vi "configureHWError.vi"(8 "error in (no error)":errorcluster, 11 "AtomChipHWC in":refnum<class "AtomChipHWC.lvclass">) -> (0 "error out":errorcluster, 2 "error":bool, 3 "AtomChipHWC out":refnum<class "AtomChipHWC.lvclass">)   [LabVIEW 2009, in "Hardware.lvlib" / "HWControllers.lvlib" / "AtomChipHWC.lvclass"]
uses:
  AtomChipHWC.lvclass
  AtomChipHWC.lvclass/AtomChipHWC.ctl
  Channels/Digital/DigitalOutput.lvclass
  Channels/VoltOutput/AnalogOutput.lvclass
  Channels/DDSOutput/Generic/DDSOutput.lvclass
  Network Controllers/CameraNetworkController/CameraNetworkController.lvclass
  HWController.lvclass
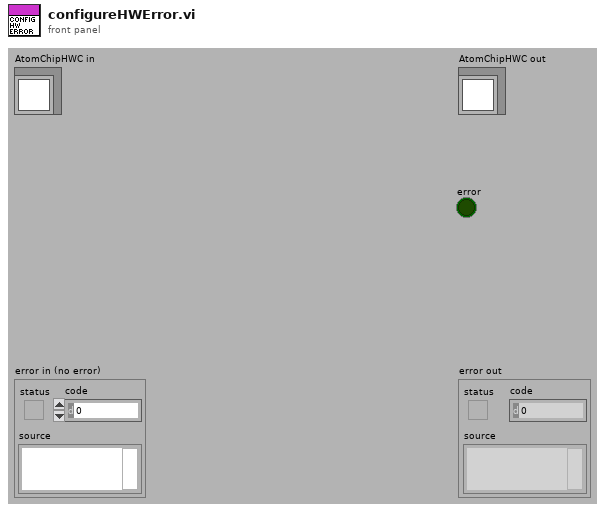
[diagram p1: front panel]
types:
  T1 = enum16{"Ready", "Compiling", "Configured", "Running", "Stopping", "Unresolved Error"}
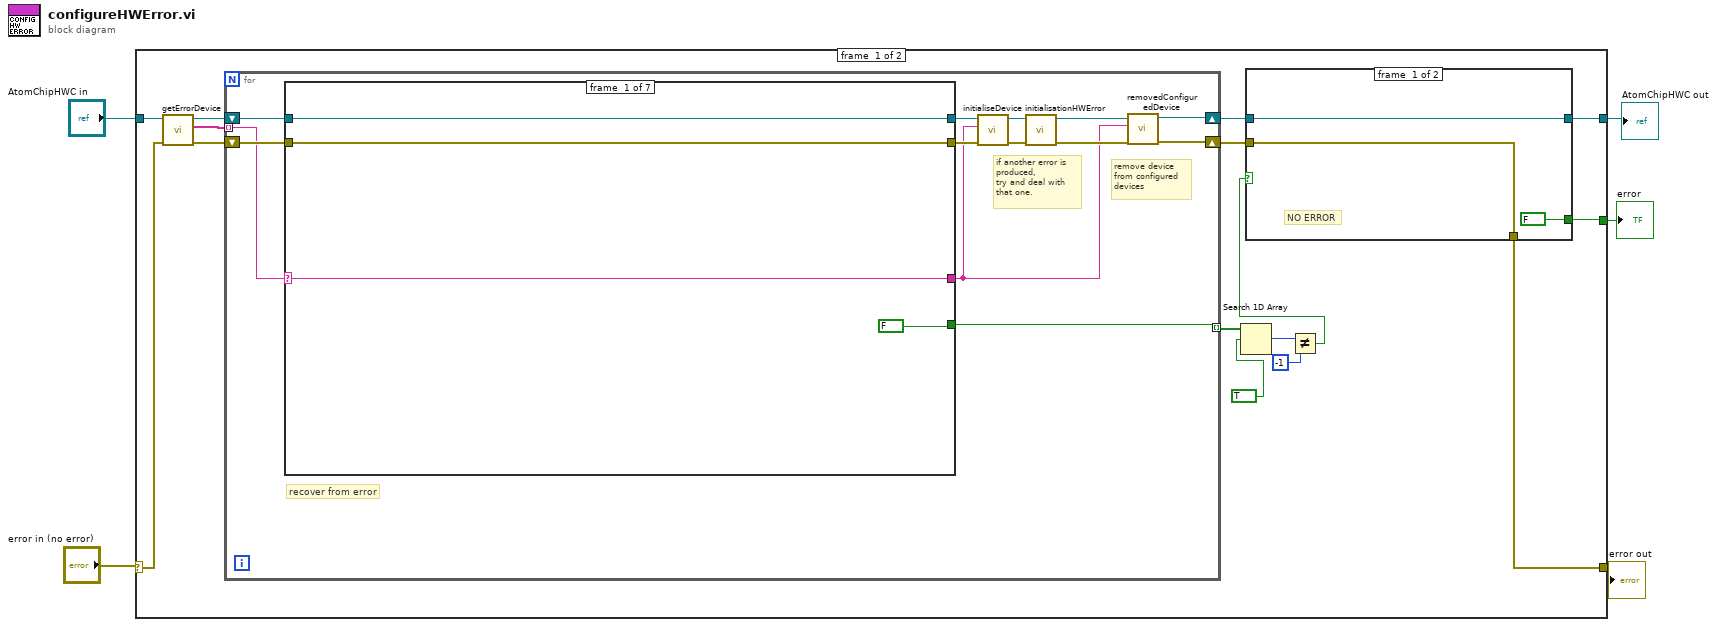
[diagram p0: block diagram]
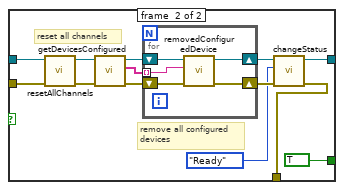
[diagram p2: hidden frame]
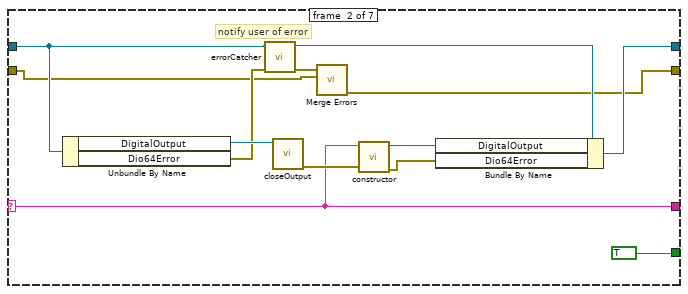
[diagram p3: hidden frame]
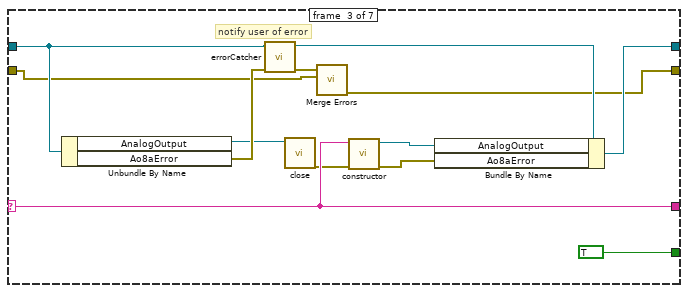
[diagram p4: hidden frame]
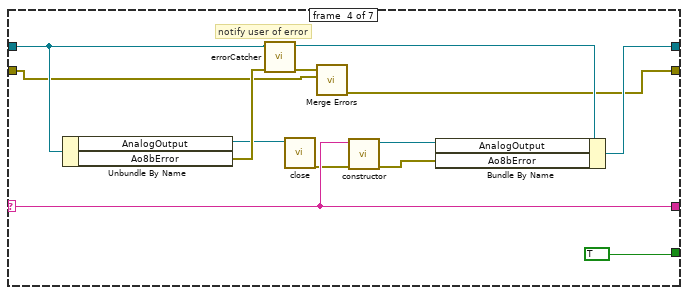
[diagram p5: hidden frame]
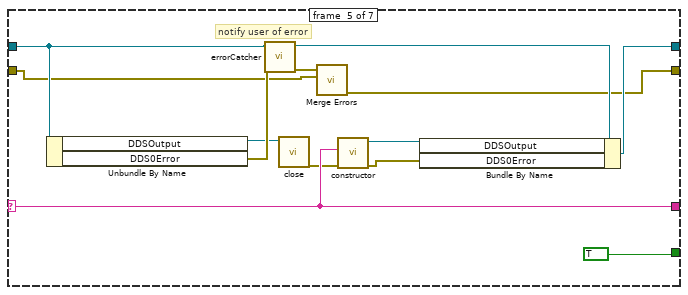
[diagram p6: hidden frame]
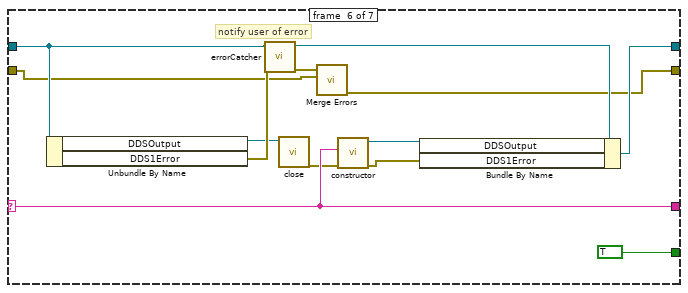
[diagram p7: hidden frame]
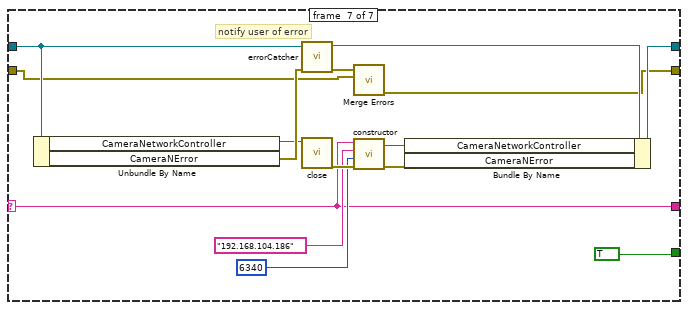
[diagram p8: hidden frame]
diagram:
  n1 = case shown="No Error" "error in (no error)" {
    selector: "error in (no error)" -> [w19 w139]
    tunnel: "AtomChipHWC in" -> [w20 w140]
    tunnel: [w12 w140] -> w3
    tunnel: [w13 w139] -> w2
    tunnel: [w11 _] -> w1
    frame #0 {
      n2 = call "getErrorDevice.vi"("error in (no error)"=w19, "AtomChipHWC in"=w20) -> ("error out"=w16:errorcluster, "Devices"=w17:string[], "AtomChipHWC out"=w18:refnum<class "AtomChipHWC.lvclass">)  [unwired: 7 in]
      n3 = for {
        tunnel: w17 -> [w52] mode=indexing
        shift-right: [w46] -> w15
        shift-left: w18 -> [w54]
        shift-right: [w45] -> w14
        shift-left: w16 -> [w53]
        tunnel: [w42] -> w10 mode=indexing
        # "remove device\nfrom configured\ndevices"
        # "if another error is\nproduced,\ntry and deal with\nthat one."
        # "recover from error"
        n4 = case shown="\"Ao8a\"" w52 {
          selector: w52 -> [w56 w60 w76 w89 w100 w113 w125]
          tunnel: w54 -> [w58 w67 w84 w97 w110 w123 w138]
          tunnel: [w58 w62 w79 w92 w105 w118 w133] -> w47
          tunnel: [w57 w61 w78 w91 w104 w117 w132] -> w44
          tunnel: w53 -> [w57 w63 w80 w93 w106 w119 w134]
          tunnel: [w56 w60 w76 w89 w100 w113 w125] -> w43
          tunnel: [FALSE TRUE TRUE TRUE TRUE TRUE TRUE] -> w42
          frame #0 {
          }
          frame #1 {
            # "notify user of error"
            n5 = Unbundle By Name(w67) -> ("DigitalOutput"=w71:refnum<class "DigitalOutput.lvclass">, "Dio64Error"=w65:errorcluster)
            n6 = call-dynamic "errorCatcher.vi"("error in (no error)"=w65, "HWController in"=w67) -> ("error out"=w64:errorcluster, "HWController out"=w66:refnum<class "AtomChipHWC.lvclass">)  [unwired: 8 in]
            n7 = call-dynamic "closeOutput.vi"("DigitalOutput in"=w71) -> ("error out"=w70:errorcluster)  [unwired: 10 in]
            n8 = call <vilib>:"Merge Errors.vi"("error in 2 (no error)"=w63, "error in 1 (no error)"=w64) -> ("error out"=w61:errorcluster)  [unwired: 5 in]
            n9 = call "constructor.vi"("error in (no error)"=w70, "deviceName"=w60) -> ("error out"=w68:errorcluster, "DigitalOutput out"=w69:refnum<class "DigitalOutput.lvclass">)  [unwired: 8 in]
            n10 = Bundle By Name(cluster=w66, "DigitalOutput"=w69, "Dio64Error"=w68) -> (w62:refnum<class "AtomChipHWC.lvclass">)
          }
          frame #2 {
            # "notify user of error"
            n11 = Unbundle By Name(w84) -> ("AnalogOutput"=w77:refnum<class "AnalogOutput.lvclass">, "Ao8aError"=w82:errorcluster)
            n12 = call-dynamic "errorCatcher.vi"("error in (no error)"=w82, "HWController in"=w84) -> ("error out"=w81:errorcluster, "HWController out"=w83:refnum<class "AtomChipHWC.lvclass">)  [unwired: 8 in]
            n13 = call-dynamic "close.vi"("AnalogOutput in"=w77) -> ("error out"=w75:errorcluster)  [unwired: 10 in]
            n14 = call <vilib>:"Merge Errors.vi"("error in 2 (no error)"=w80, "error in 1 (no error)"=w81) -> ("error out"=w78:errorcluster)  [unwired: 5 in]
            n15 = call "constructor.vi"("error in (no error)"=w75, "deviceName"=w76) -> ("error out"=w73:errorcluster, "AnalogOutput out"=w74:refnum<class "AnalogOutput.lvclass">)  [unwired: 8 in]
            n16 = Bundle By Name(cluster=w83, "AnalogOutput"=w74, "Ao8aError"=w73) -> (w79:refnum<class "AtomChipHWC.lvclass">)
          }
          frame #3 {
            # "notify user of error"
            n17 = Unbundle By Name(w97) -> ("AnalogOutput"=w90:refnum<class "AnalogOutput.lvclass">, "Ao8bError"=w95:errorcluster)
            n18 = call-dynamic "errorCatcher.vi"("error in (no error)"=w95, "HWController in"=w97) -> ("error out"=w94:errorcluster, "HWController out"=w96:refnum<class "AtomChipHWC.lvclass">)  [unwired: 8 in]
            n19 = call-dynamic "close.vi"("AnalogOutput in"=w90) -> ("error out"=w88:errorcluster)  [unwired: 10 in]
            n20 = call <vilib>:"Merge Errors.vi"("error in 2 (no error)"=w93, "error in 1 (no error)"=w94) -> ("error out"=w91:errorcluster)  [unwired: 5 in]
            n21 = call "constructor.vi"("error in (no error)"=w88, "deviceName"=w89) -> ("error out"=w86:errorcluster, "AnalogOutput out"=w87:refnum<class "AnalogOutput.lvclass">)  [unwired: 8 in]
            n22 = Bundle By Name(cluster=w96, "AnalogOutput"=w87, "Ao8bError"=w86) -> (w92:refnum<class "AtomChipHWC.lvclass">)
          }
          frame #4 {
            # "notify user of error"
            n23 = Unbundle By Name(w110) -> ("DDSOutput"=w103:refnum<class "DDSOutput.lvclass">, "DDS0Error"=w108:errorcluster)
            n24 = call-dynamic "errorCatcher.vi"("error in (no error)"=w108, "HWController in"=w110) -> ("error out"=w107:errorcluster, "HWController out"=w109:refnum<class "AtomChipHWC.lvclass">)  [unwired: 8 in]
            n25 = call-dynamic "close.vi"("DDSOutput in"=w103) -> ("error out"=w99:errorcluster)  [unwired: 10 in]
            n26 = call <vilib>:"Merge Errors.vi"("error in 2 (no error)"=w106, "error in 1 (no error)"=w107) -> ("error out"=w104:errorcluster)  [unwired: 5 in]
            n27 = call "constructor.vi"("error in (no error)"=w99, "device"=w100) -> ("error out"=w101:errorcluster, "DDSOutput out"=w102:refnum<class "DDSOutput.lvclass">)  [unwired: 8 in]
            n28 = Bundle By Name(cluster=w109, "DDSOutput"=w102, "DDS0Error"=w101) -> (w105:refnum<class "AtomChipHWC.lvclass">)
          }
          frame #5 {
            # "notify user of error"
            n29 = Unbundle By Name(w123) -> ("DDSOutput"=w116:refnum<class "DDSOutput.lvclass">, "DDS1Error"=w121:errorcluster)
            n30 = call-dynamic "errorCatcher.vi"("error in (no error)"=w121, "HWController in"=w123) -> ("error out"=w120:errorcluster, "HWController out"=w122:refnum<class "AtomChipHWC.lvclass">)  [unwired: 8 in]
            n31 = call-dynamic "close.vi"("DDSOutput in"=w116) -> ("error out"=w112:errorcluster)  [unwired: 10 in]
            n32 = call <vilib>:"Merge Errors.vi"("error in 2 (no error)"=w119, "error in 1 (no error)"=w120) -> ("error out"=w117:errorcluster)  [unwired: 5 in]
            n33 = call "constructor.vi"("error in (no error)"=w112, "device"=w113) -> ("error out"=w114:errorcluster, "DDSOutput out"=w115:refnum<class "DDSOutput.lvclass">)  [unwired: 8 in]
            n34 = Bundle By Name(cluster=w122, "DDSOutput"=w115, "DDS1Error"=w114) -> (w118:refnum<class "AtomChipHWC.lvclass">)
          }
          frame #6 {
            # "notify user of error"
            n35 = Unbundle By Name(w138) -> ("CameraNetworkController"=w131:refnum<class "CameraNetworkController.lvclass">, "CameraNError"=w136:errorcluster)
            n36 = call-dynamic "errorCatcher.vi"("error in (no error)"=w136, "HWController in"=w138) -> ("error out"=w135:errorcluster, "HWController out"=w137:refnum<class "AtomChipHWC.lvclass">)  [unwired: 8 in]
            n37 = call "close.vi"("CameraNetworkController in"=w131) -> ("error out"=w128:errorcluster)  [unwired: 9 in, 1 out]
            n38 = call <vilib>:"Merge Errors.vi"("error in 2 (no error)"=w134, "error in 1 (no error)"=w135) -> ("error out"=w132:errorcluster)  [unwired: 5 in]
            n39 = call "constructor.vi"("error in (no error)"=w128, "remote port"=u16 6340, "remote address"="192.168.104.186", "camera"=w125) -> ("error out"=w129:errorcluster, "CameraNetworkController out"=w130:refnum<class "CameraNetworkController.lvclass">)  [unwired: 6 in]
            n40 = Bundle By Name(cluster=w137, "CameraNetworkController"=w130, "CameraNError"=w129) -> (w133:refnum<class "AtomChipHWC.lvclass">)
          }
        }
        n41 = call "initialiseDevice.vi"("error in (no error)"=w44, "deviceName"=w43, "AtomChipHWC in"=w47) -> ("error out"=w50:errorcluster, "AtomChipHWC out"=w51:refnum<class "AtomChipHWC.lvclass">)  [unwired: 7 in]
        n42 = call-dynamic "initialisationHWError.vi"("error in (no error)"=w50, "AtomChipHWC in"=w51) -> ("error out"=w48:errorcluster, "AtomChipHWC out"=w49:refnum<class "AtomChipHWC.lvclass">)  [unwired: 8 in]
        n43 = call-dynamic "removedConfiguredDevice.vi"("error in (no error)"=w48, "device"=w43, "HWController in"=w49) -> ("error out"=w45:errorcluster, "HWController out"=w46:refnum<class "AtomChipHWC.lvclass">)  [unwired: 7 in]
      }
      n44 = Search 1D Array(1D array=w10, element=TRUE) -> (index of element=w8:i32)  [unwired: 1 in]
      n45 = Not Equal?(x=w8, y=-1) -> (x != y?=w6:bool)
      n46 = case shown="True" w6 {
        tunnel: w15 -> [w23 w36]
        tunnel: w14 -> [w22 w35]
        tunnel: [w22 w25] -> w13
        tunnel: [w23 w27] -> w12
        tunnel: [FALSE TRUE] -> w11
        frame #0 {
          # "NO ERROR"
        }
        frame #1 {
          # "remove all configured\ndevices"
          # "reset all channels"
          n47 = call-dynamic "resetAllChannels.vi"("error in (no error)"=w35, "AtomChipHWC in"=w36) -> ("error out"=w33:errorcluster, "AtomChipHWC out"=w34:refnum<class "AtomChipHWC.lvclass">)  [unwired: 8 in]
          n48 = call "getDevicesConfigured.vi"("error in (no error)"=w33, "HWController.lvclass in"=w34) -> ("error out"=w31:errorcluster, "devicesConfigured"=w30:string[], "HWController.lvclass out"=w32:refnum<class "AtomChipHWC.lvclass">)  [unwired: 7 in]
          n49 = for {
            shift-right: [w40] -> w28
            shift-left: w32 -> [w41]
            shift-right: [w38] -> w26
            shift-left: w31 -> [w39]
            tunnel: w30 -> [w37] mode=indexing
            n50 = call-dynamic "removedConfiguredDevice.vi"("error in (no error)"=w39, "device"=w37, "HWController in"=w41) -> ("error out"=w38:errorcluster, "HWController out"=w40:refnum<class "AtomChipHWC.lvclass">)  [unwired: 7 in]
          }
          n51 = call "changeStatus.vi"("error in (no error)"=w26, "status"=T1."Ready", "HWController in"=w28) -> ("error out"=w25:errorcluster, "HWController out"=w27:refnum<class "AtomChipHWC.lvclass">)  [unwired: 7 in]
        }
      }
    }
    frame #1 {
    }
  }
  "error out" <- w2
  "AtomChipHWC out" <- w3
  "error" <- w1
